vi "EXDIR-YAML_DetermineArraySize.vi"(10 "start":i32, 11 "ENTIRE Array of YAML Lines":string[](array[string])) -> (2 "indent size of this array":i32, 3 "Length":i32)   [LabVIEW 2016]
panel:
  out "element":string
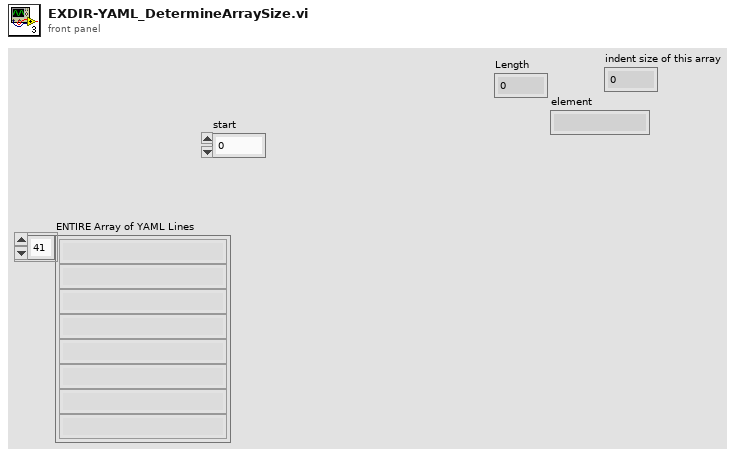
[diagram p1: front panel]
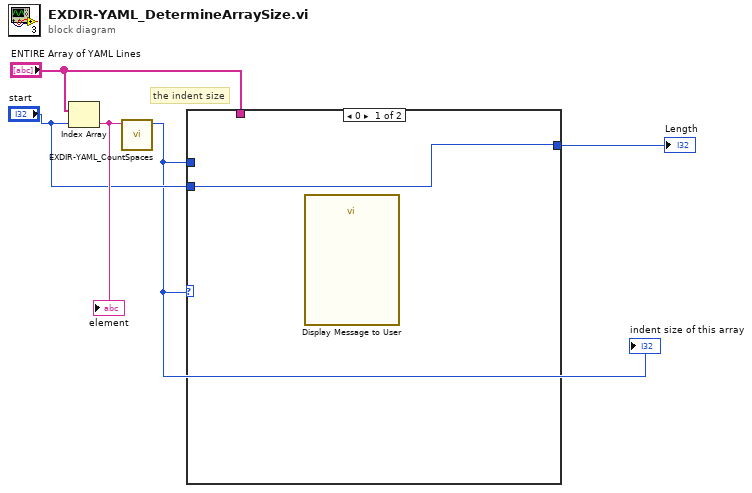
[diagram p0: block diagram]
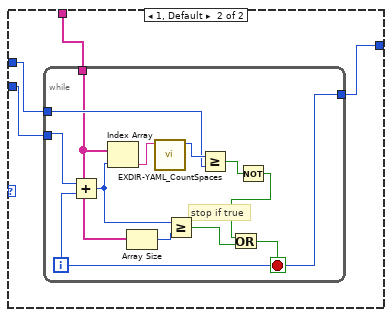
[diagram p2: hidden frame]
diagram:
  # "the indent size"
  n1 = Index Array(array="ENTIRE Array of YAML Lines", index="start") -> (element=w5:string)
  "element" <- w5
  n2 = call "EXDIR-YAML_CountSpaces.vi"("String"=w5) -> ("Numeric"=w1:i32)  [unwired: 10 in]
  "indent size of this array" <- w1
  n3 = case shown="0" w1 {
    tunnel: "ENTIRE Array of YAML Lines" -> [_ w10]
    tunnel: "start" -> [w6 w9]
    tunnel: w1 -> [_ w8]
    tunnel: [w6 w7] -> w2
    frame 0 {
      n4 = call "Display Message to User"() -> ()  [unwired: 10 in, 2 out]
    }
    frame 1, Default {
      n5 = while {
        tunnel: w10 -> [w18]
        tunnel: w9 -> [w22]
        tunnel: w8 -> [w19]
        tunnel: [w11] -> w7
        i -> [w11]
        stop <- w12 stop-if-true
        # "stop if true"
        n6 = Add(x=w22, y=w11) -> (x+y=w16:i32)
        n7 = Index Array(array=w18, index=w16) -> (element=w21:string)
        n8 = Array Size(array=w18) -> (size(s)=w17:i32)
        n9 = call "EXDIR-YAML_CountSpaces.vi"("String"=w21) -> ("Numeric"=w20:i32)  [unwired: 10 in]
        n10 = Greater Or Equal?(x=w16, y=w17) -> (x >= y?=w14:bool)
        n11 = Greater Or Equal?(x=w20, y=w19) -> (x >= y?=w15:bool)
        n12 = Not(x=w15) -> (.not. x?=w13:bool)
        n13 = Or(x=w13, y=w14) -> (x .or. y?=w12:bool)
      }
    }
  }
  "Length" <- w2
